vi "Debounce.vi"(1 "Input":bool=TRUE, 2 "Num samples":i32) -> (0 "Output":bool=TRUE)   [LabVIEW 2016]
panel:
  in  "counter":i32
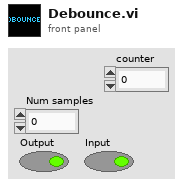
[diagram p1: front panel]
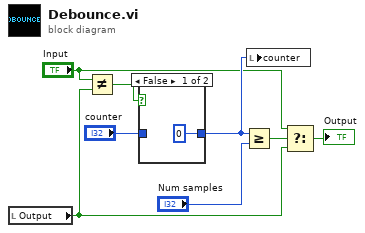
[diagram p0: block diagram]
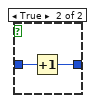
[diagram p2: hidden frame]
diagram:
  n1 = local read "Output"() -> (w2:bool)
  n2 = Not Equal?(x="Input", y=w2) -> (x != y?=w8:bool)
  n3 = case shown="False" w8 {
    tunnel: "counter" -> [_ w11]
    tunnel: [0 w10] -> w6
    frame False {
    }
    frame True {
      n4 = Increment(x=w11) -> (x+1=w10:i32)
    }
  }
  n5 = Greater Or Equal?(x=w6, y="Num samples") -> (x >= y?=w4:bool)
  n6 = local write "counter"(w6) -> ()
  n7 = Select(t="Input", s=w4, f=w2) -> (s? t:f=→"Output":bool)
